vi "Loop unroll.vi"(1 "Loop":string="filename\nloop(3){pump /1Q #query pump\npump /1? #report absolute plunger position\npump /1?6 #report valve position}\nloop(3){pump /2Q #query pump}", 2 "Offset of inner loop end":i32, 3 "Offset of inner loop start":i32) -> (0 "Unrolled loop":string="filename\npump /1Q #query pump\npump /1? #report absolute plunger position\npump /1?6 #report valve position\rpump /1Q #query pump\npump /1? #report absolute plunger position\npump /1?6 #report valve position\rpump /1Q #query pump\npump /1? #report absolute plunger position\npump /1?6 #report valve position\npump /2Q #query pump\rpump /2Q #query pump\rpump /2Q #query pump")   [LabVIEW 2019]
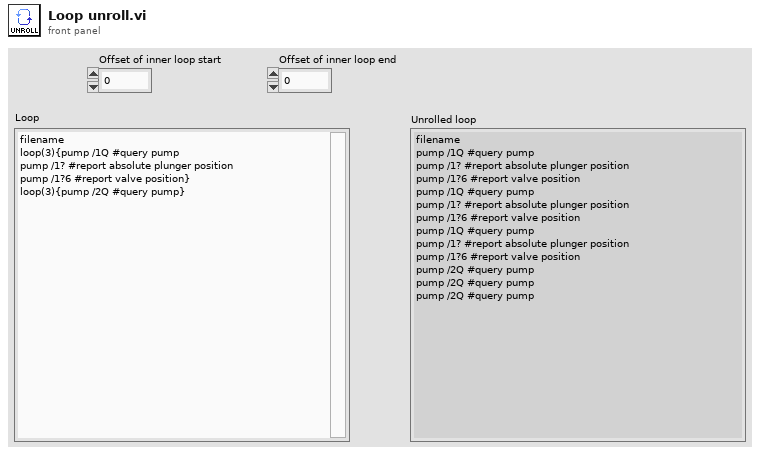
[diagram p1: front panel]
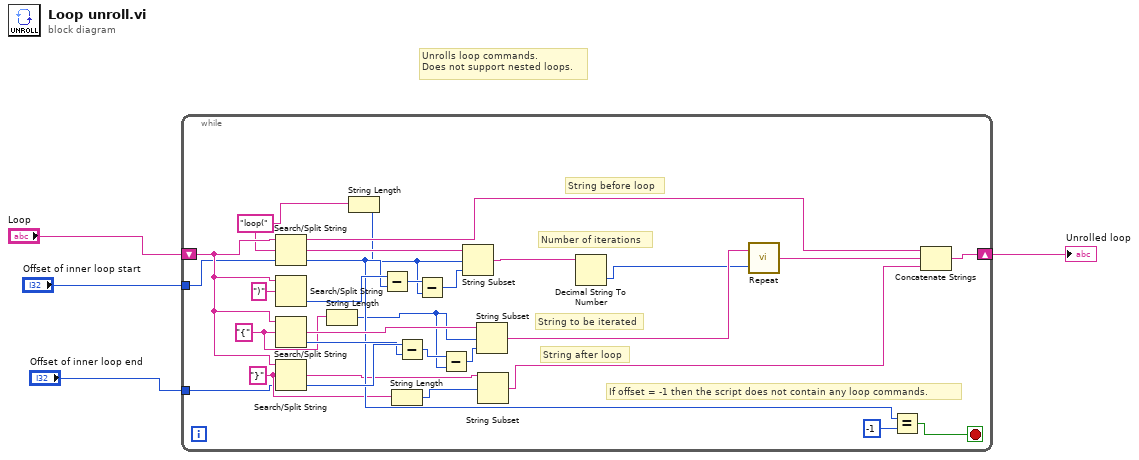
[diagram p0: block diagram]
diagram:
  # "Unrolls loop commands.\nDoes not support nested loops."
  n1 = while {
    shift-right: [w34] -> w3
    shift-left: "Loop" -> [w16]
    tunnel: "Offset of inner loop start" -> [w6]
    tunnel: "Offset of inner loop end" -> [w5]
    stop <- w17 stop-if-true
    w7 = "}" ("search string/char (-)")
    w9 = "{" ("search string/char (-)")
    w12 = "loop(" ("search string/char (-)")
    # "String after loop"
    # "String before loop"
    # "Number of iterations"
    # "String to be iterated"
    # "If offset = -1 then the script does not contain any loop commands."
    n2 = Search/Split String(string=w16, search string/char (-)=w12, offset (0)=w6) -> (substring before match=w31:string, match + rest of string=w29:string, offset of match=w18:i32)
    n3 = Search/Split String(string=w16, search string/char (-)=")") -> (offset of match=w30:i32)  [unwired: 1 in, 2 out]
    n4 = Search/Split String(string=w16, search string/char (-)=w9) -> (match + rest of string=w26:string, offset of match=w27:i32)  [unwired: 1 in, 1 out]
    n5 = Search/Split String(string=w16, search string/char (-)=w7, offset (0)=w5) -> (match + rest of string=w14:string, offset of match=w28:i32)  [unwired: 1 out]
    n6 = String Length(string=w9) -> (length=w10:i32)
    n7 = String Length(string=w12) -> (length=w11:i32)
    n8 = Subtract(x=w30, y=w18) -> (x-y=w22:i32)
    n9 = String Length(string=w7) -> (length=w8:i32)
    n10 = Subtract(x=w28, y=w27) -> (x-y=w25:i32)
    n11 = Subtract(x=w22, y=w11) -> (x-y=w21:i32)
    n12 = Subtract(x=w25, y=w10) -> (x-y=w24:i32)
    n13 = String Subset(string=w29, offset (0)=w11, length (rest)=w21) -> (substring=w20:string)
    n14 = String Subset(string=w26, offset (0)=w10, length (rest)=w24) -> (substring=w23:string)
    n15 = String Subset(string=w14, offset (0)=w8) -> (substring=w13:string)  [unwired: 1 in]
    n16 = Decimal String To Number(string=w20) -> (number=w19:i32)  [unwired: 2 in, 1 out]
    n17 = call "Repeat.vi"("Iterations"=w19, "Script"=w23) -> ("Output"=w33:string)
    n18 = Equal?(x=w18, y=-1) -> (x = y?=w17:bool)
    n19 = Concatenate Strings(w31, w33, w13) -> (w34:string)
  }
  "Unrolled loop" <- w3
